vi "Pre Launch Init.vi"(11 "Aumentar_contador in":refnum<class "Aumentar_contador.lvclass">) -> (0 "error out":errorcluster, 3 "Aumentar_contador out":refnum<class "Aumentar_contador.lvclass">)   [LabVIEW 2019, in "Aumentar_contador.lvlib" / "Aumentar_contador.lvclass"]
doc: "(<B>Filename</B>: Actor Framework.lvlib:Actor.lvclass:Pre Launch Init.vi)\n\nDefines behavior that occurs after the Launch Nested Actor method is invoked but before the actor's Actor Core method begins running.\n\nBy default, this method does nothing. A descendant class may override it to define behavior."
uses:
  Aumentar_contador.lvclass
  Aumentar_contador.lvclass/Aumentar_contador.ctl
  <vilib>/ActorFramework/Actor/Actor.lvclass
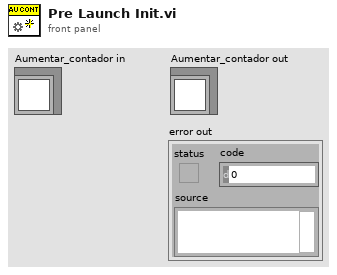
[diagram p1: front panel]
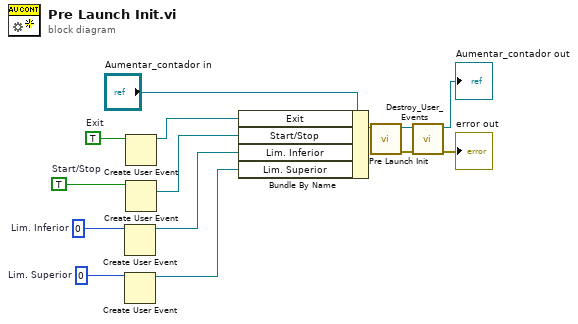
[diagram p0: block diagram]
diagram:
  w3 = u8 0  # Lim. Superior
  w4 = u8 0  # Lim. Inferior
  w13 = TRUE  # Start/Stop
  w14 = TRUE  # Exit
  n1 = Create User Event(user event datatype=w4) -> (user event=w2:refnum<user-event>)  [unwired: 1 in, 1 out]
  n2 = Create User Event(user event datatype=w3) -> (user event=w1:refnum<user-event>)  [unwired: 1 in, 1 out]
  n3 = Create User Event(user event datatype=w14) -> (user event=w10:refnum<user-event>)  [unwired: 1 in, 1 out]
  n4 = Create User Event(user event datatype=w13) -> (user event=w5:refnum<user-event>)  [unwired: 1 in, 1 out]
  n5 = Bundle By Name(cluster="Aumentar_contador in", "Exit"=w10, "Start/Stop"=w5, "Lim. Inferior"=w2, "Lim. Superior"=w1) -> (w11:refnum<class "Aumentar_contador.lvclass">)
  n6 = call-parent "Pre Launch Init.vi"("Actor in"=w11) -> ("error out"=w9:errorcluster, "Actor out"=w8:refnum<class "Aumentar_contador.lvclass">)  [unwired: 9 in]
  n7 = call "Destroy_User_Events.vi"("error in (no error)"=w9, "Aumentar_contador in"=w8) -> ("error out"=→"error out":errorcluster, "Aumentar_contador out"=→"Aumentar_contador out":refnum<class "Aumentar_contador.lvclass">)  [unwired: 8 in]
